vi "AgKs_SpecAn_Capture.vi"(5 "Error In":errorcluster) -> (19 "Error Out":errorcluster)   [LabVIEW 2015]
doc: "AgKs SpecAn Screen Capture is a simple screen capture tool for most Agilent PSA/ESA and Keysight MXA/PXA spectrum analyzers"
uses:
  Controls/FGV Action SpecAn Model.ctl
  Controls/SpecAn Cluster.ctl
panel:
  in  "Noise Source":bool
  in  "Frequency Ref In":i32(ring) items=["Internal", "External"]
  in  "Marker Peak":bool
  in  "Cont Update":bool
  in  "Preamp State":bool
  in  "Avg State":bool
  in  "VBW Auto/Man":bool=TRUE
  in  "RBW Auto/Man":bool=TRUE
  in  "RBW (Hz)":i32=30000000 min=10 step=1 format="%#.6p"
  in  "VBW (Hz)":i32=30000000 min=10 step=1 format="%#.6p"
  in  "Avg Count":u32=10 min=1 max=5000 step=1
  in  "Ref Level (dBm)":dbl=10.0 min=-120.0 max=30.0 step=1.0 format="%#.2f"
  in  "Span (Hz)":dbl=5000000.0 min=10.0 max=30000000000.0 step=1.0 format="%#.6p"
  in  "Center Freq (Hz)":dbl=1000000000.0 min=10.0 max=30000000000.0 step=1.0 format="%#.6p"
  in  "Attenuation (dB)":dbl=20.0 format="%#.2f"
  in  "VISA Handle":refnum<visa-resource-name>="SpecAn"
  in  "Capture":bool
  in  "Auto Align Enable":bool
  in  "Zoom Factor":sgl min=0 max=10 step=0.1
  in  "Secured View":bool
  in  "Full Screen":bool
  out "Pic":picture
  out "PIC_PATH":path
  out "INI PATH":path
  out "State":string="Close GUI"
  out "ZoomFactor_Hi":dbl
  out "ZoomFactor_Lo":dbl
  in  "Save Image?":bool
  # "Note:\n\nPSA screen dim: 640x480\nPSA: Use Zoom Factor = 0\n\nPXA screen dim: 1024x768\nPXA: Use Zoom Factor = 0.7"
  # "Agilent/Keysight PSA/ESA/MXA/PXA Screen Capture Tool"
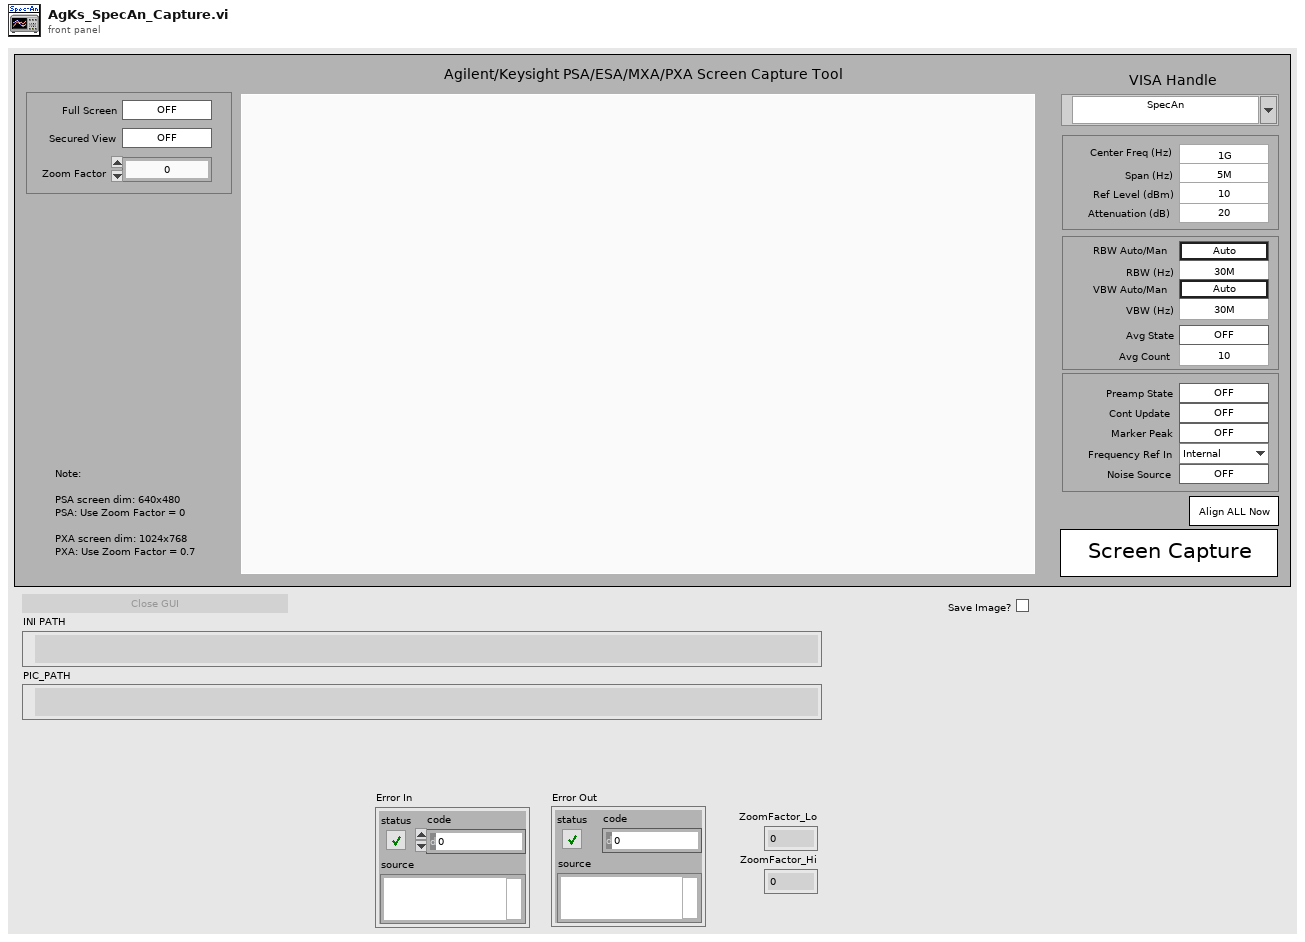
[diagram p1: front panel]
types:
  T1 = cluster{"SA VISA":refnum<visa-resource-name>, "PATH":path, "This VI":refnum<vi>, "VI Name":string}
  T2 = typedef "SpecAn Cluster.ctl" = cluster{"Span (Hz)":dbl, "Center Freq (Hz)":dbl, "Mode":i32, "Frequency Ref In":i32, "Trace Type":i32, "Trace":i32, "Enable Trace Update":bool, "Enable Trace Display":bool, "Manual VBW":i32, "Auto VBW":bool, "Manual RBW":i32, "Auto RBW":bool, "Amplitude Units":i32, "Reference Level":dbl, "Reference Level Offset":dbl, "Averaging On/Off":i32, "Marker Type":i32, "Readout":i32, "Active Marker":i32, "Auto Align Enable":enum16{"Disable", "Enable"}}
  T3 = typedef "FGV Action SpecAn Model.ctl" = enum16{"Get", "Set"}
  T4 = typedef "imagedata.ctl" = cluster{"image type":i32, "image depth":i32, "image":u8[], "mask":u8[], "colors":u32[], "Rectangle":cluster{"left":i16, "top":i16, "right":i16, "bottom":i16}}
  T5 = typedef "SpecAn Model.ctl" = enum16{"E4440", "N9030"}
  T6 = enum32{"Invalid", "Standard", "Closed", "Hidden", "Minimized", "Maximized"}
  T7 = enum32{"invalid app kind", "Development System", "Run Time System", "Student Edition", "Embedded LabVIEW", "Evaluation", "Custom"}
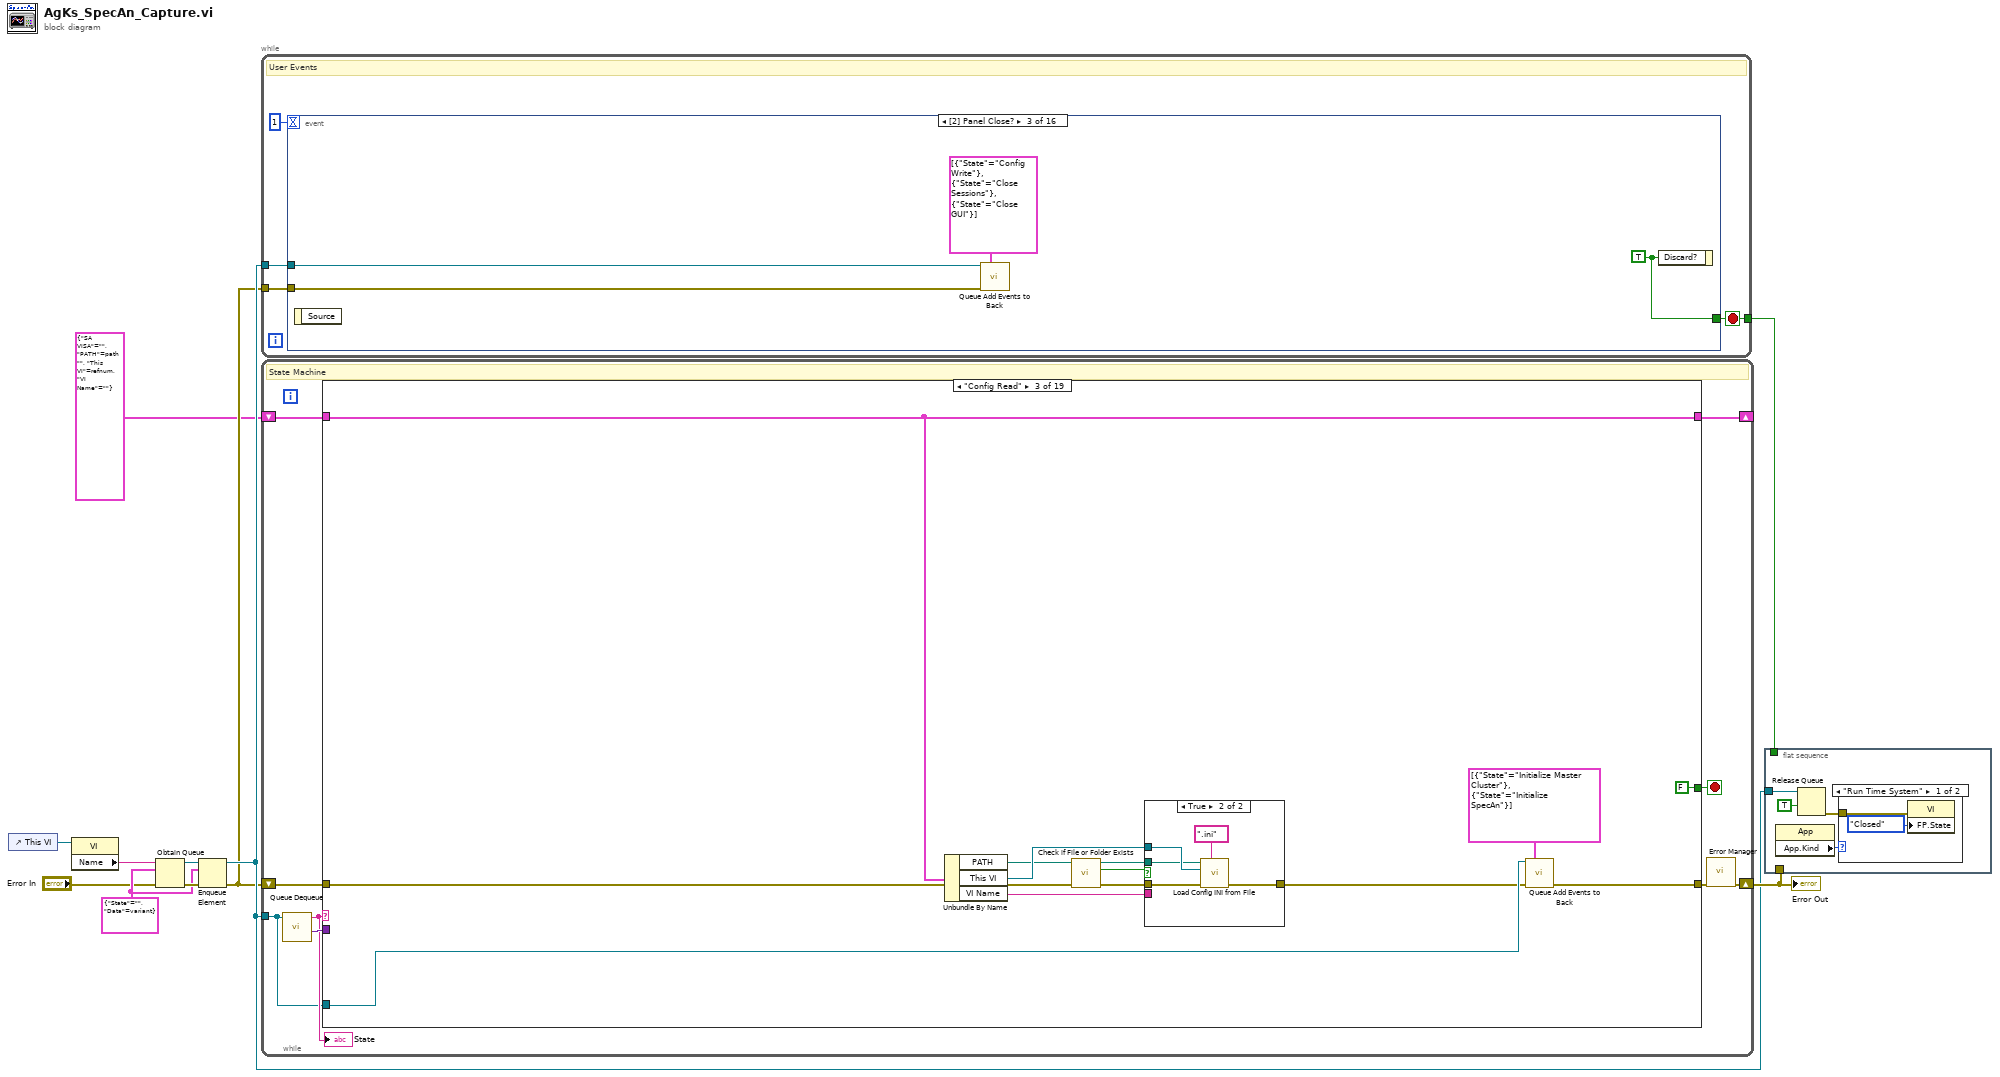
[diagram p0: block diagram]
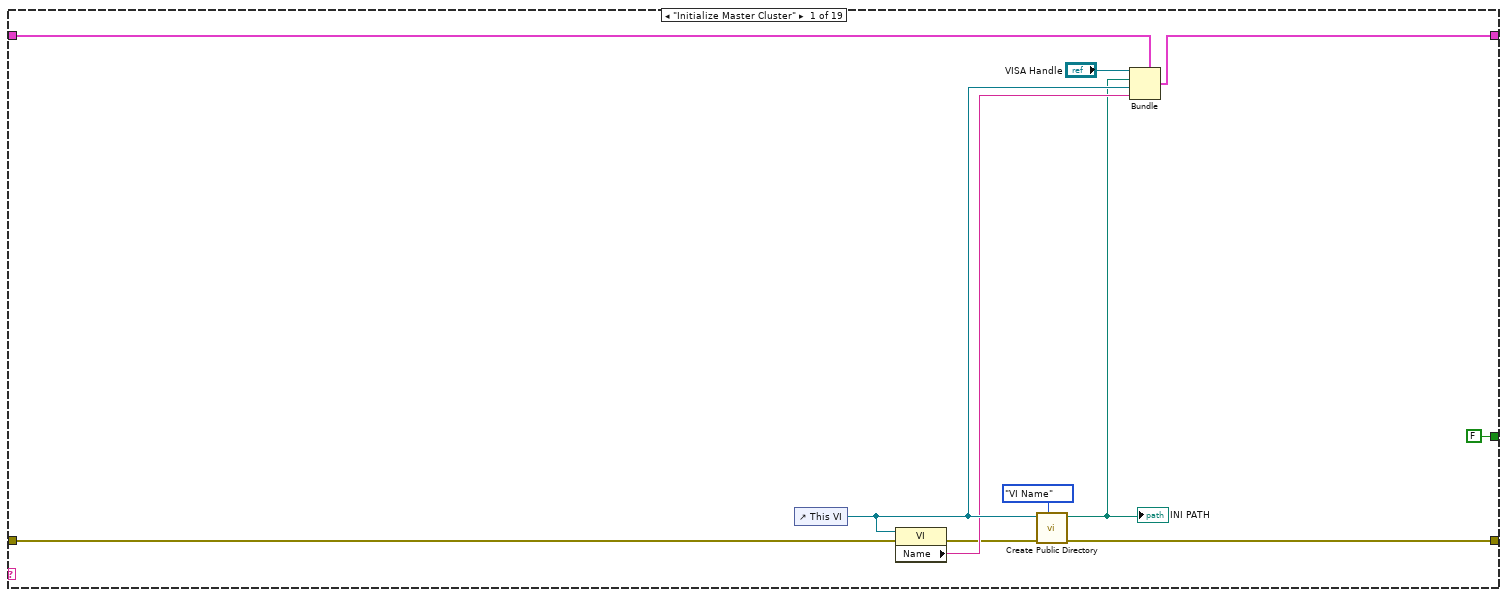
[diagram p3: hidden frame]
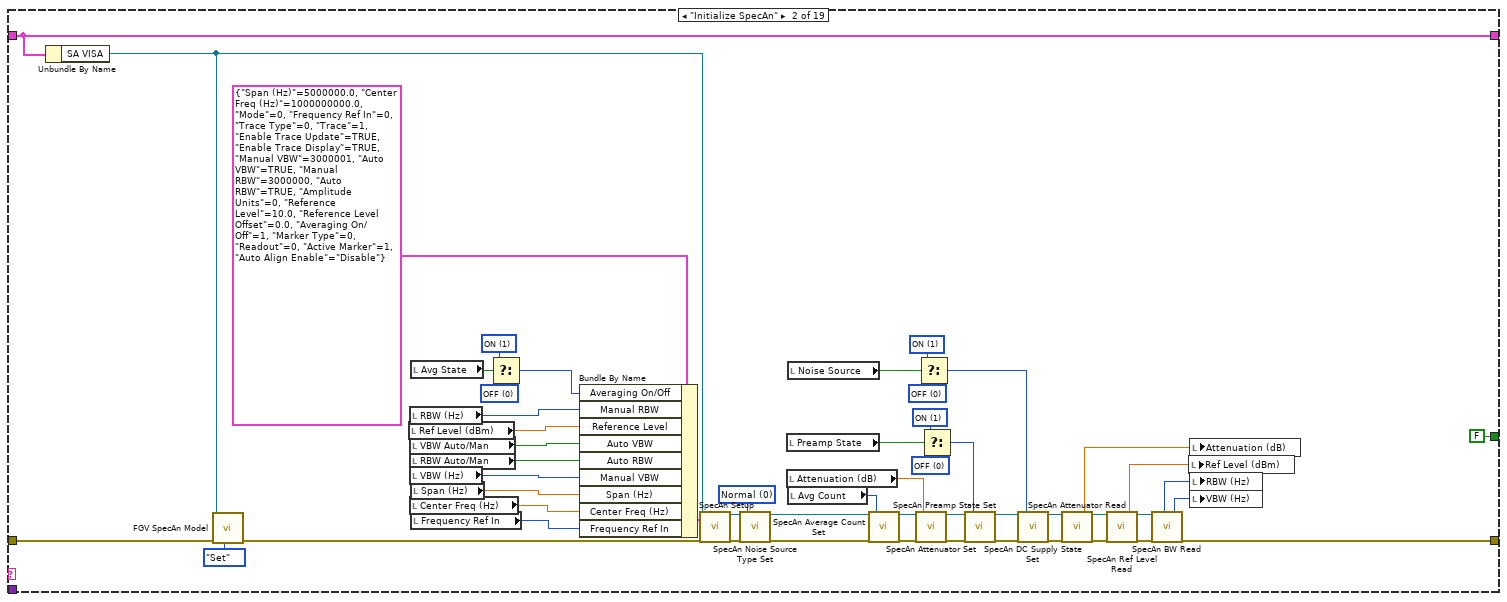
[diagram p4: hidden frame]
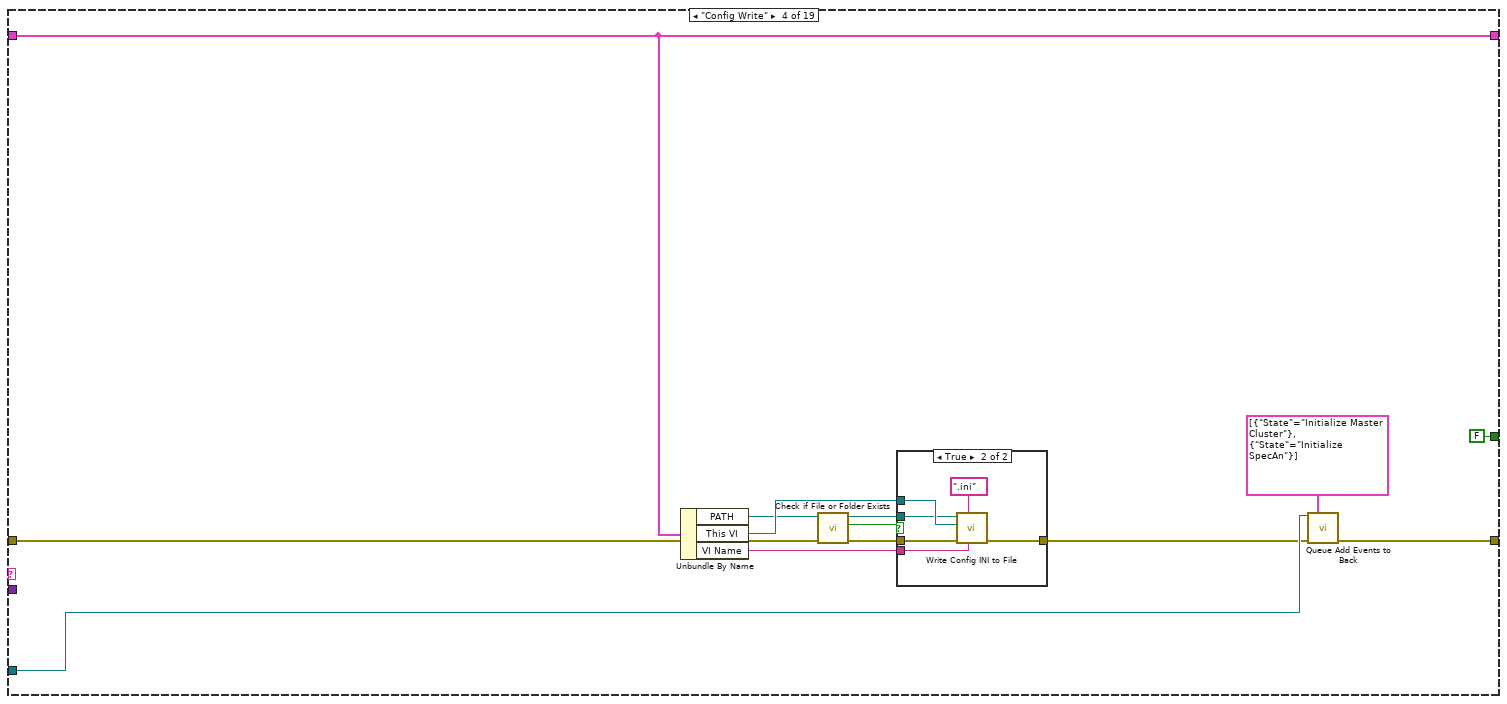
[diagram p6: hidden frame]
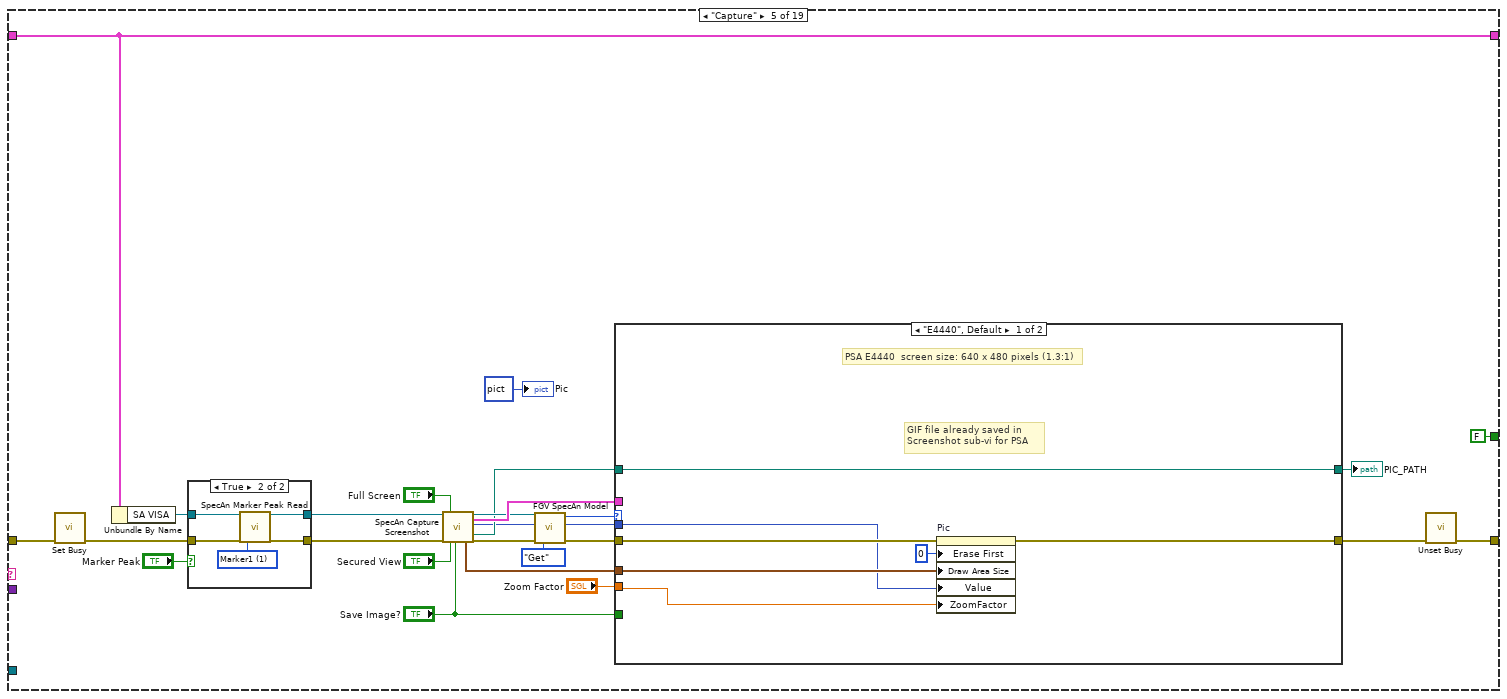
[diagram p8: hidden frame]
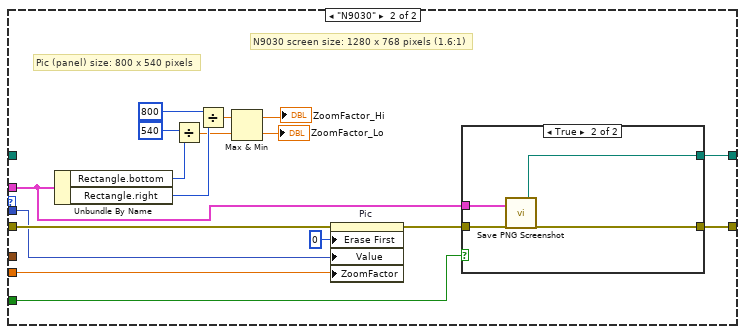
[diagram p9: hidden frame]
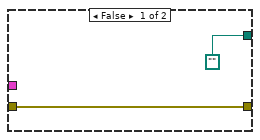
[diagram p10: hidden frame]
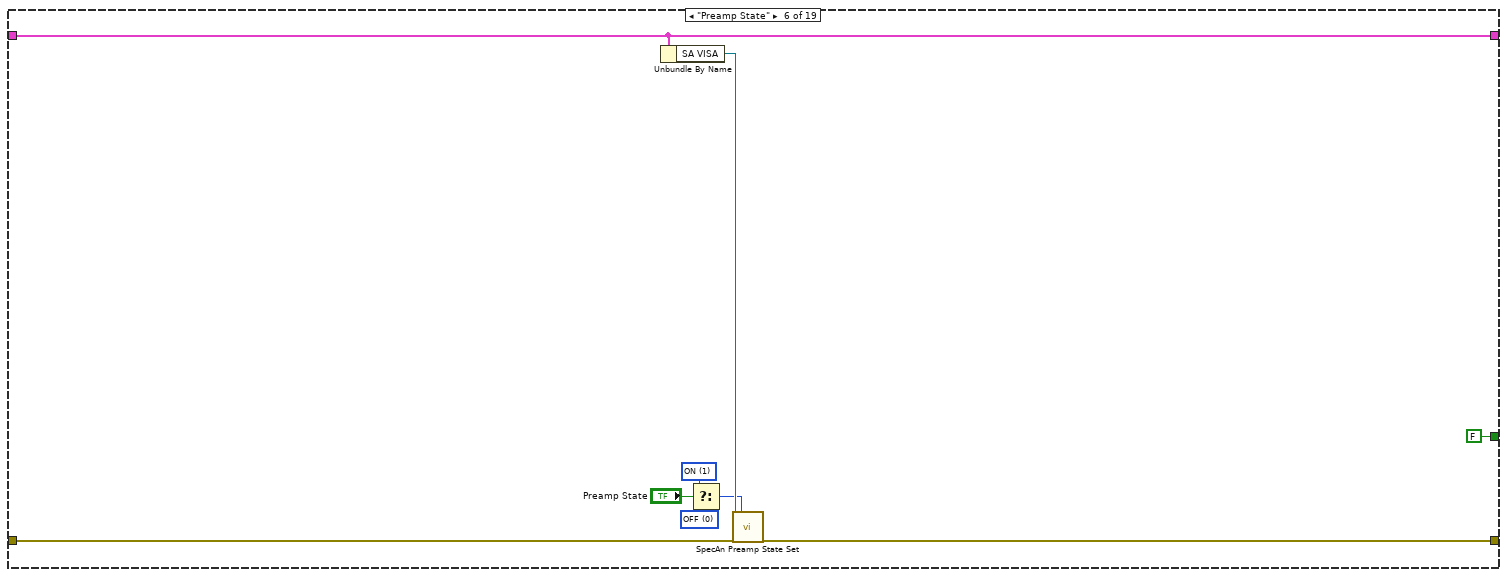
[diagram p12: hidden frame]
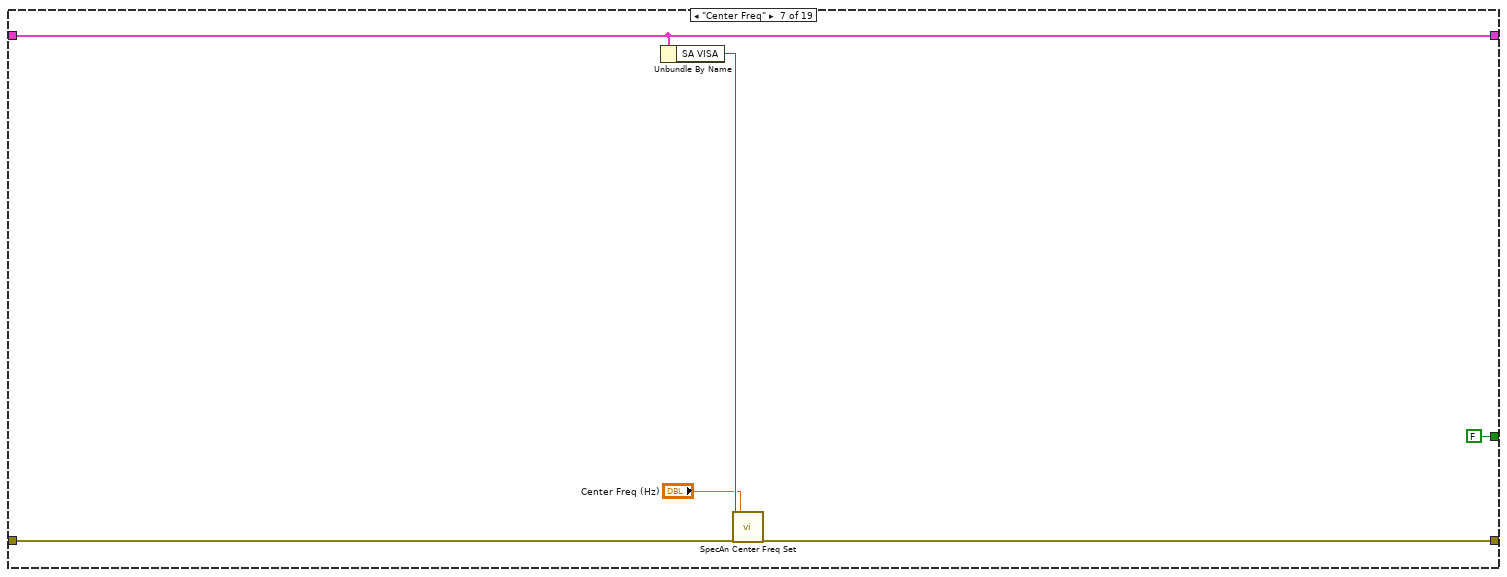
[diagram p13: hidden frame]
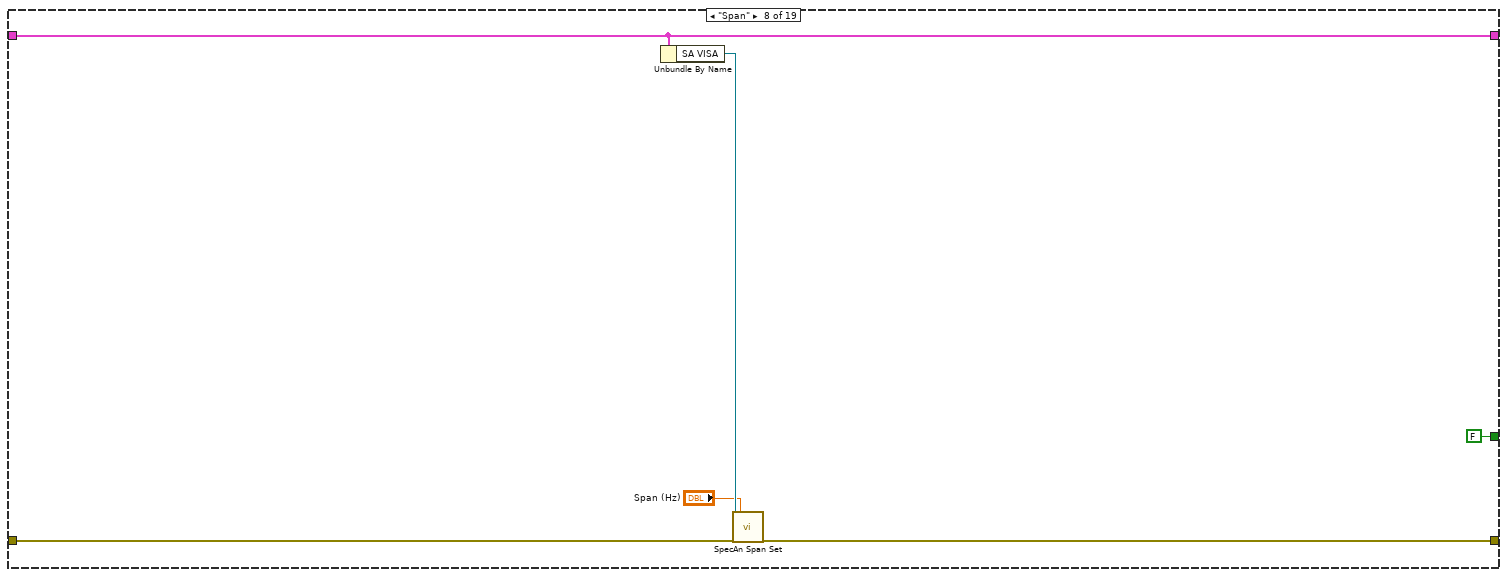
[diagram p14: hidden frame]
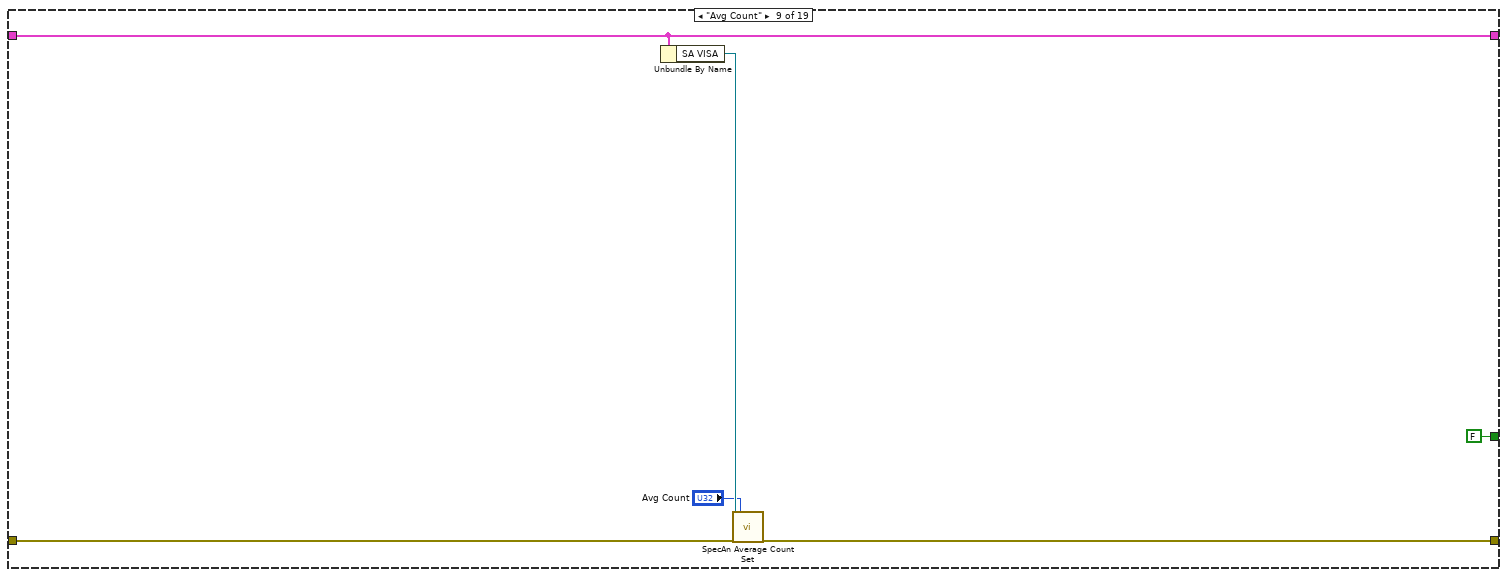
[diagram p15: hidden frame]
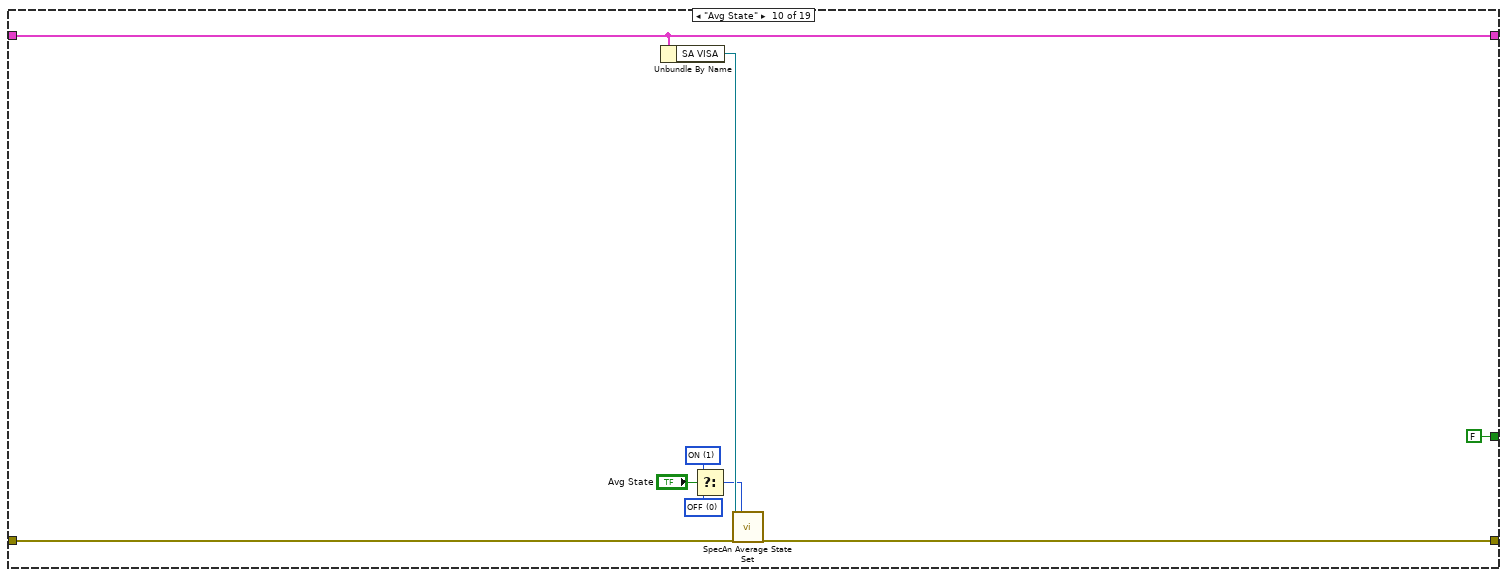
[diagram p16: hidden frame]
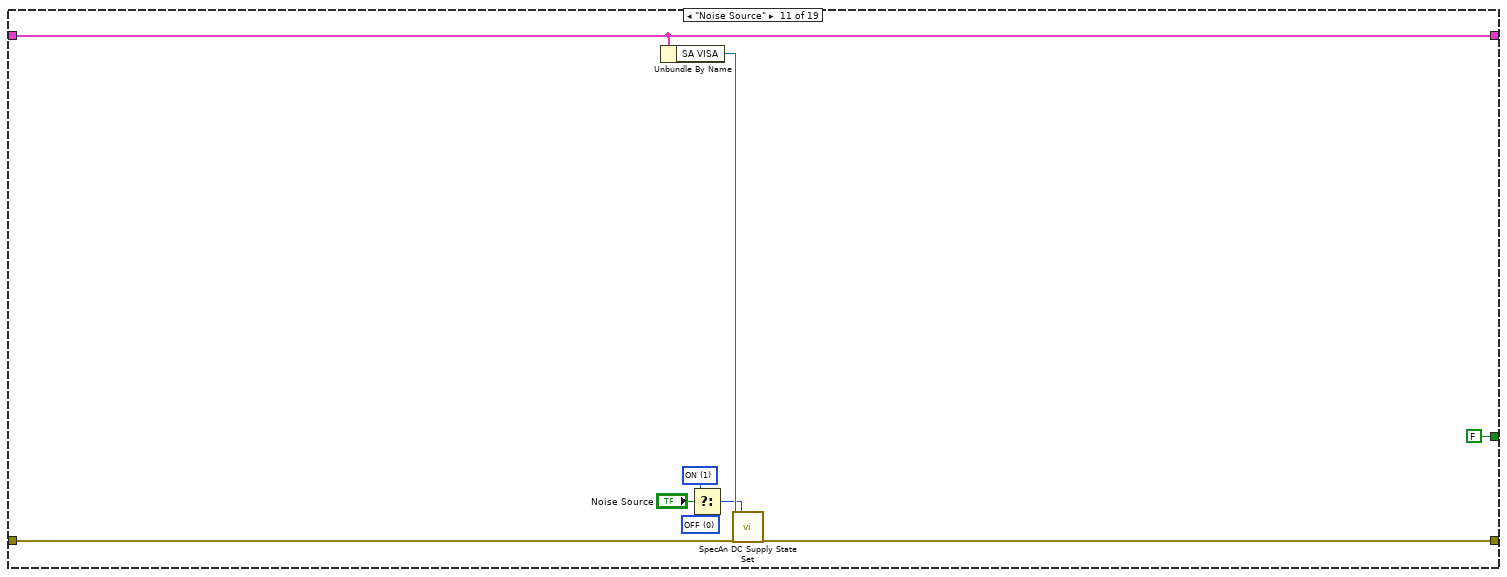
[diagram p17: hidden frame]
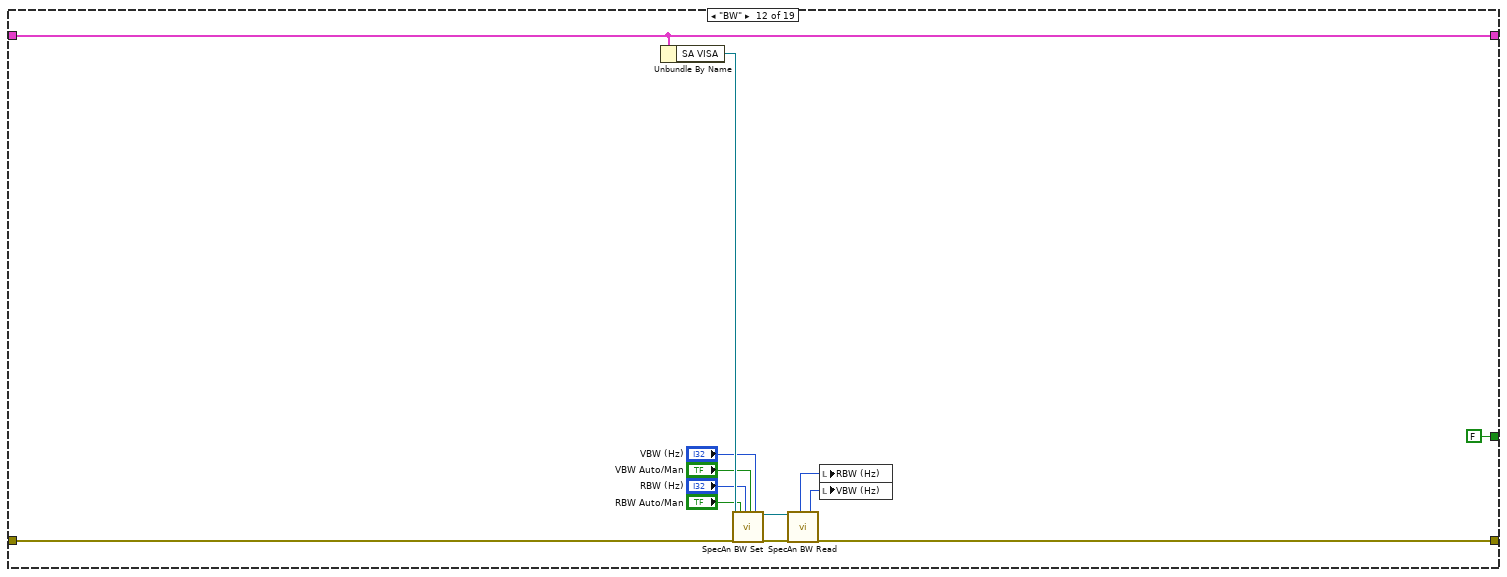
[diagram p18: hidden frame]
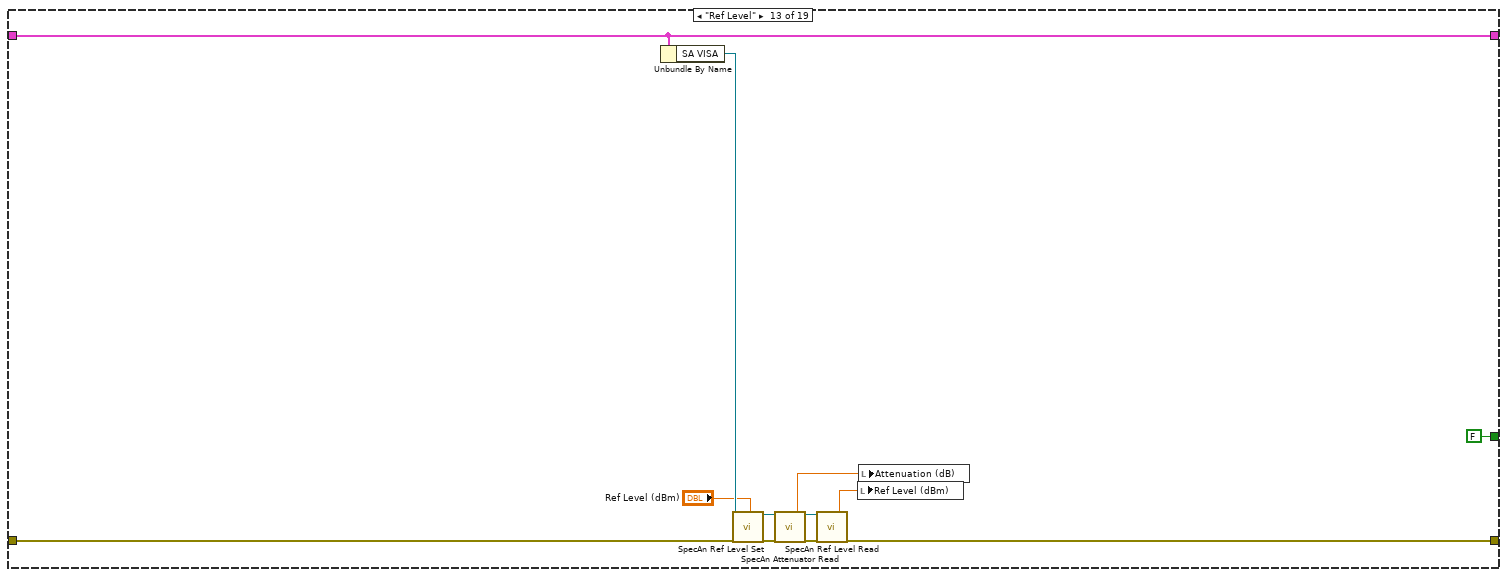
[diagram p19: hidden frame]
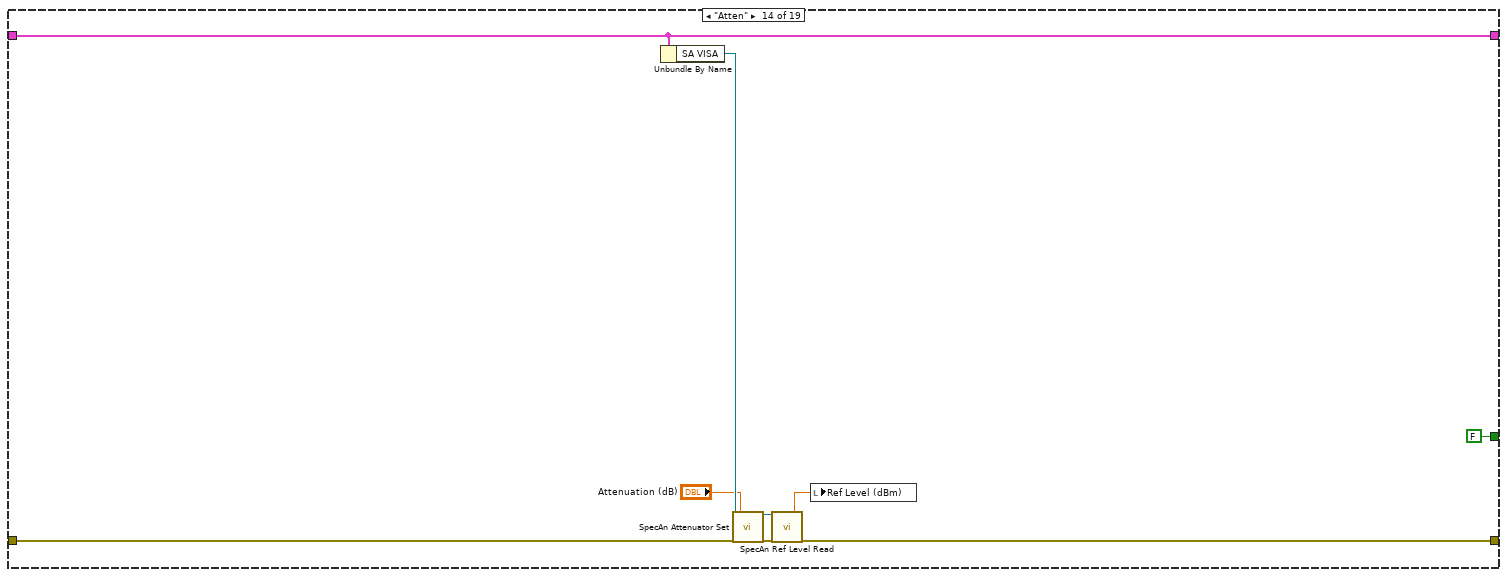
[diagram p20: hidden frame]
diagram:
  w7 = cluster{"State":string, "Data":variant} {"State"="", "Data"=variant} ("Cluster")
  n1 = control-ref of="This VI"() -> (w4:refnum<vi>)
  n2 = property class="VI"(reference=w4) -> ("Name"=w1:string)  [unwired: 1 in, 2 out]
  n3 = Obtain Queue(name (unnamed)=w1, element data type=w7, error in (no error)="Error In") -> (queue out=w10:refnum<queue>, error out=w11:errorcluster)  [unwired: 2 in, 1 out]
  n4 = Enqueue Element(queue=w10, element=w7, error in (no error)=w11) -> (queue out=w6:refnum<queue>, error out=w3:errorcluster)  [unwired: 1 in, 1 out]
  n5 = while {
    tunnel: w6 -> [w15]
    tunnel: [w14] -> w9
    tunnel: w3 -> [w12]
    stop <- w14 stop-if-true
    # "User Events"
    n6 = event shown="[2] Panel Close?" {
      selector: _ -> [_ _ _ _ _ _ _ _ _ _ _ _ _ _ _ _]
      dyn-events: _ -> [_ _ _ _ _ _ _ _ _ _ _ _ _ _ _ _]
      timeout: 1 -> [_ _ _ _ _ _ _ _ _ _ _ _ _ _ _ _]
      tunnel: w15 -> [w18 w25 w33 w36 w39 w42 w45 w48 w51 w54 w57 w60 w63 w66 w69 w72]
      tunnel: [FALSE ("Abort?") FALSE ("Abort?") w32 _ _ _ _ _ _ _ _ _ _ _ _ _] -> w14
      tunnel: w12 -> [w17 w23 w31 w35 w38 w41 w44 w47 w50 w53 w56 w59 w62 w65 w68 _]
      event Timeout {
        n7 = event-data() -> ()  [unwired: 1 in, 1 out]
        n8 = First Call?() -> (First Call?: T/F=w16:bool)
        n9 = case shown="True" w16 {
          tunnel: w18 -> [_ w21]
          tunnel: w17 -> [_ w20]
          frame False {
          }
          frame True {
            n10 = call "Queue Add Events to Back.vi"("Queue In"=w21, "State Array"=cluster{"State":string}[] [{"State"="Config Read"}], "Error In"=w20) -> ()  [unwired: 11 in, 2 out]
          }
        }
      }
      event Menu Selection (User) {
        n11 = event-data() -> ("ItemTag"=w27:string, "ItemPath"=w26:string)  [unwired: 1 in]
        n12 = case shown="Default" w26 {
          tunnel: w25 -> [w30]
          tunnel: w27 -> [w29]
          tunnel: w23 -> [w28]
          frame Default {
            n13 = call "Queue Add Events to Back with Data.vi"("Queue In"=w30, "Error In"=w28, "State"=w29) -> ()  [unwired: 15 in, 2 out]
          }
        }
      }
      event Panel Close? {
        w32 = TRUE ("Discard?")
        n14 = event-data() -> ()  [unwired: 1 in, 1 out]
        n15 = call "Queue Add Events to Back.vi"("Queue In"=w33, "State Array"=cluster{"State":string}[] [{"State"="Config Write"}, {"State"="Close Sessions"}, {"State"="Close GUI"}], "Error In"=w31) -> ()  [unwired: 11 in, 2 out]
        n16 = event-data("Discard?"=w32) -> ()  [unwired: 1 in, 1 out]
      }
      event "VISA Handle": Value Change {
        n17 = event-data() -> ()  [unwired: 1 in, 2 out]
        n18 = call "Queue Add Events to Back.vi"("Queue In"=w36, "State Array"=cluster{"State":string}[] [{"State"="Close Sessions"}, {"State"="Master Cluster"}], "Error In"=w35) -> ()  [unwired: 11 in, 2 out]
      }
      event "Preamp State": Value Change {
        n19 = event-data() -> ()  [unwired: 1 in, 2 out]
        n20 = call "Queue Add Events to Back.vi"("Queue In"=w39, "State Array"=cluster{"State":string}[] [{"State"="Preamp State"}], "Error In"=w38) -> ()  [unwired: 11 in, 2 out]
      }
      event "Center Freq (Hz)": Value Change {
        n21 = event-data() -> ()  [unwired: 1 in, 2 out]
        n22 = call "Queue Add Events to Back.vi"("Queue In"=w42, "State Array"=cluster{"State":string}[] [{"State"="Center Freq"}], "Error In"=w41) -> ()  [unwired: 11 in, 2 out]
      }
      event "Span (Hz)": Value Change {
        n23 = event-data() -> ()  [unwired: 1 in, 2 out]
        n24 = call "Queue Add Events to Back.vi"("Queue In"=w45, "State Array"=cluster{"State":string}[] [{"State"="Span"}], "Error In"=w44) -> ()  [unwired: 11 in, 2 out]
      }
      event "Avg Count": Value Change {
        n25 = event-data() -> ()  [unwired: 1 in, 2 out]
        n26 = call "Queue Add Events to Back.vi"("Queue In"=w48, "State Array"=cluster{"State":string}[] [{"State"="Avg Count"}], "Error In"=w47) -> ()  [unwired: 11 in, 2 out]
      }
      event "Avg State": Value Change {
        n27 = event-data() -> ()  [unwired: 1 in, 2 out]
        n28 = call "Queue Add Events to Back.vi"("Queue In"=w51, "State Array"=cluster{"State":string}[] [{"State"="Avg State"}], "Error In"=w50) -> ()  [unwired: 11 in, 2 out]
      }
      event "VBW (Hz)", "VBW Auto/Man", "RBW (Hz)", "RBW Auto/Man": Value Change {
        n29 = event-data() -> ()  [unwired: 1 in, 2 out]
        n30 = call "Queue Add Events to Back.vi"("Queue In"=w54, "State Array"=cluster{"State":string}[] [{"State"="BW"}], "Error In"=w53) -> ()  [unwired: 11 in, 2 out]
      }
      event "Ref Level (dBm)": Value Change {
        n31 = event-data() -> ()  [unwired: 1 in, 2 out]
        n32 = call "Queue Add Events to Back.vi"("Queue In"=w57, "State Array"=cluster{"State":string}[] [{"State"="Ref Level"}], "Error In"=w56) -> ()  [unwired: 11 in, 2 out]
      }
      event "Attenuation (dB)": Value Change {
        n33 = event-data() -> ()  [unwired: 1 in, 2 out]
        n34 = call "Queue Add Events to Back.vi"("Queue In"=w60, "State Array"=cluster{"State":string}[] [{"State"="Atten"}], "Error In"=w59) -> ()  [unwired: 11 in, 2 out]
      }
      event "Frequency Ref In": Value Change {
        n35 = event-data() -> ()  [unwired: 1 in, 2 out]
        n36 = call "Queue Add Events to Back.vi"("Queue In"=w63, "State Array"=cluster{"State":string}[] [{"State"="Freq Ref"}], "Error In"=w62) -> ()  [unwired: 11 in, 2 out]
      }
      event "Auto Align Enable": Value Change {
        n37 = event-data() -> ()  [unwired: 1 in, 2 out]
        n38 = call "Queue Add Events to Back.vi"("Queue In"=w66, "State Array"=cluster{"State":string}[] [{"State"="Auto Align"}], "Error In"=w65) -> ()  [unwired: 11 in, 2 out]
      }
      event "Noise Source": Value Change {
        n39 = event-data() -> ()  [unwired: 1 in, 2 out]
        n40 = call "Queue Add Events to Back.vi"("Queue In"=w69, "State Array"=cluster{"State":string}[] [{"State"="Noise Source"}], "Error In"=w68) -> ()  [unwired: 11 in, 2 out]
      }
      event "Capture": Value Change {
        n41 = event-data() -> ("NewVal"=w71:bool)  [unwired: 1 in]
        n42 = case shown="True" w71 {
          tunnel: w72 -> [_ w73]
          frame False {
          }
          frame True {
            n43 = call "Queue Add Events to Back.vi"("Queue In"=w73, "State Array"=cluster{"State":string}[] [{"State"="Capture"}]) -> ()  [unwired: 12 in, 2 out]
          }
        }
      }
    }
  }
  n44 = while {
    shift-right: [w83] -> w8
    shift-left: w3 -> [w75]
    shift-right: [w79] -> _
    shift-left: T1 {"SA VISA"="", "PATH"=path "", "This VI"=refnum, "VI Name"=""} -> [w80]
    tunnel: w6 -> [w76]
    stop <- w81 stop-if-true
    # "State Machine"
    n45 = call "Queue Dequeue.vi"("Queue In"=w76) -> ("Data"=w78:variant, "State"=w77:string)  [unwired: 8 in, 1 out]
    "State" <- w77
    n46 = case shown="\"Config Read\"" w77 {
      tunnel: [w91 w144 w158 w177 w187 w248 w259 w265 w271 w280 w289 w296 w307 w319 w329 w334 w348 w358 w364] -> w82
      tunnel: w76 -> [_ _ w159 w178 _ _ _ _ _ _ _ _ _ _ _ _ w347 _ _]
      tunnel: [FALSE FALSE FALSE FALSE FALSE FALSE FALSE FALSE FALSE FALSE FALSE FALSE FALSE FALSE FALSE FALSE FALSE FALSE TRUE] -> w81
      tunnel: w80 -> [w92 w96 w154 w173 w209 w254 w261 w267 w273 w282 w291 w304 w316 w325 w332 w338 w350 w361 w362]
      tunnel: [w94 w96 w154 w173 w209 w254 w261 w267 w273 w282 w291 w304 w316 w325 w332 w338 w350 w361 w362] -> w79
      tunnel: w78 -> [_ _ _ _ _ _ _ _ _ _ _ _ _ _ _ _ _ _ _]
      tunnel: w75 -> [w85 w145 w151 w170 w203 w255 w260 w266 w272 w281 w290 w303 w315 w323 w330 w337 w349 w360 w364]
      frame "Initialize Master Cluster" {
        n47 = control-ref of="This VI"() -> (w90:refnum<vi>)
        n48 = property class="VI"(reference=w90, error in=w85) -> (error out=w84:errorcluster, "Name"=w89:string)  [unwired: 1 out]
        n49 = call "Create Public Directory.vi"("Name Type"=enum16{"VI Name", "Custom Name"}."VI Name", "error in (no error)"=w84, "Caller_VI"=w90) -> ("error out"=w91:errorcluster, "PATH"=w87:path)  [unwired: 7 in]
        "INI PATH" <- w87
        n50 = Bundle(cluster=w92, "SA VISA"="VISA Handle", "PATH"=w87, "This VI"=w90, "VI Name"=w89) -> (w94:T1)
      }
      frame "Initialize SpecAn" {
        w104 = 0 items=["OFF", "ON"] ("State")
        w103 = 1 items=["OFF", "ON"] ("State")
        w109 = 0 items=["Normal", "SNS"] ("Type")
        w128 = 0 items=["OFF", "ON"] ("Averaging On/Off")
        w127 = 1 items=["OFF", "ON"] ("Averaging On/Off")
        w131 = 1 items=["OFF", "ON"] ("State")
        w132 = 0 items=["OFF", "ON"] ("State")
        n51 = Unbundle By Name(w96) -> ("SA VISA"=w95:refnum<visa-resource-name>)
        n52 = call "FGV SpecAn Model.vi"("Action"=FGV_Action_SpecAn_Model."Set", "Error In"=w145, "VISA In"=w95) -> ("Error Out"=w138:errorcluster)  [unwired: 4 in, 1 out]
        n53 = local read "Ref Level (dBm)"() -> (w125:dbl)
        n54 = local read "RBW (Hz)"() -> (w119:i32)
        n55 = local read "VBW Auto/Man"() -> (w124:bool)
        n56 = local read "RBW Auto/Man"() -> (w123:bool)
        n57 = local read "VBW (Hz)"() -> (w120:i32)
        n58 = local read "Center Freq (Hz)"() -> (w121:dbl)
        n59 = local read "Avg State"() -> (w129:bool)
        n60 = local read "Span (Hz)"() -> (w122:dbl)
        n61 = local read "Frequency Ref In"() -> (w110:i32)
        n62 = Select(t=w127, s=w129, f=w128) -> (s? t:f=w126:i32)
        n63 = Bundle By Name(cluster=T2 {"Span (Hz)"=5000000.0, "Center Freq (Hz)"=1000000000.0, "Mode"=0, "Frequency Ref In"=0, "Trace Type"=0, "Trace"=1, "Enable Trace Update"=TRUE, "Enable Trace Display"=TRUE, "Manual VBW"=3000001, "Auto VBW"=TRUE, "Manual RBW"=3000000, "Auto RBW"=TRUE, "Amplitude Units"=0, "Reference Level"=10.0, "Reference Level Offset"=0.0, "Averaging On/Off"=1, "Marker Type"=0, "Readout"=0, "Active Marker"=1, "Auto Align Enable"=enum."Disable"} ("SpecAn Cluster"), "Averaging On/Off"=w126, "Manual RBW"=w119, "Reference Level"=w125, "Auto VBW"=w124, "Auto RBW"=w123, "Manual VBW"=w120, "Span (Hz)"=w122, "Center Freq (Hz)"=w121, "Frequency Ref In"=w110) -> (w141:T2)
        n64 = call "SpecAn Setup.vi"("VISA In"=w95, "SpecAn Cluster"=w141, "Error In"=w138) -> ("VISA Out"=w106:refnum<visa-resource-name>, "Error Out"=w108:errorcluster)  [unwired: 15 in]
        n65 = call "SpecAn Noise Source Type Set.vi"("VISA In"=w106, "Error In"=w108, "Type"=w109) -> ("VISA Out"=w105:refnum<visa-resource-name>, "Error Out"=w107:errorcluster)  [unwired: 15 in]
        n66 = local read "Preamp State"() -> (w133:bool)
        n67 = local read "Attenuation (dB)"() -> (w134:dbl)
        n68 = local read "Noise Source"() -> (w102:bool)
        n69 = local read "Avg Count"() -> (w135:u32)
        n70 = call "SpecAn Average Count Set.vi"("VISA In"=w105, "Error In"=w107, "Avg Count"=w135) -> ("VISA Out"=w139:refnum<visa-resource-name>, "Error Out"=w140:errorcluster)  [unwired: 15 in]
        n71 = call "SpecAn Attenuator Set.vi"("VISA In"=w139, "Error In"=w140, "Attenuation (dB)"=w134) -> ("VISA Out"=w136:refnum<visa-resource-name>, "Error Out"=w137:errorcluster)  [unwired: 15 in]
        n72 = Select(t=w103, s=w102, f=w104) -> (s? t:f=w101:i32)
        n73 = Select(t=w131, s=w133, f=w132) -> (s? t:f=w130:i32)
        n74 = call "SpecAn Preamp State Set.vi"("VISA In"=w136, "Error In"=w137, "State"=w130) -> ("VISA Out"=w100:refnum<visa-resource-name>, "Error Out"=w97:errorcluster)  [unwired: 15 in]
        n75 = call "SpecAn DC Supply State Set.vi"("VISA In"=w100, "Error In"=w97, "State"=w101) -> ("VISA Out"=w99:refnum<visa-resource-name>, "Error Out"=w98:errorcluster)  [unwired: 15 in]
        n76 = call "SpecAn Attenuator Read.vi"("VISA In"=w99, "Error In"=w98) -> ("Attenuation (dB)"=w112:dbl, "VISA Out"=w113:refnum<visa-resource-name>, "Error Out"=w116:errorcluster)  [unwired: 15 in]
        n77 = call "SpecAn Ref Level Read.vi"("VISA In"=w113, "Error In"=w116) -> ("Ref Level (dBm)"=w111:dbl, "VISA Out"=w114:refnum<visa-resource-name>, "Error Out"=w115:errorcluster)  [unwired: 15 in]
        n78 = call "SpecAn BW Read.vi"("VISA In"=w114, "Error In"=w115) -> ("Manual RBW"=w118:i32, "Manual VBW"=w117:i32, "Error Out"=w144:errorcluster)  [unwired: 12 in, 3 out]
        n79 = local write "Ref Level (dBm)"(w111) -> ()
        n80 = local write "Attenuation (dB)"(w112) -> ()
        n81 = local write "RBW (Hz)"(w118) -> ()
        n82 = local write "VBW (Hz)"(w117) -> ()
      }
      frame "Config Read" {
        n83 = Unbundle By Name(w154) -> ("PATH"=w149:path, "This VI"=w153:refnum<vi>, "VI Name"=w152:string)
        n84 = call <vilib>:"Check if File or Folder Exists.vi"("error in (no error)"=w151, "path"=w149) -> ("error out"=w150:errorcluster, "file or folder exists?"=w147:bool, "dup path"=w148:path)  [unwired: 7 in]
        n85 = case shown="True" w147 {
          tunnel: w150 -> [w160 w165]
          tunnel: [w160 w164] -> w155
          tunnel: w153 -> [_ w162]
          tunnel: w152 -> [_ _]
          tunnel: w148 -> [_ w161]
          frame False {
          }
          frame True {
            n86 = call "Load Config INI from File.vi"("File Type"=".ini", "Error In"=w165, "reference"=w162, "Path In"=w161) -> ("Error Out"=w164:errorcluster)  [unwired: 6 in, 1 out]
          }
        }
        n87 = call "Queue Add Events to Back.vi"("Queue In"=w159, "State Array"=cluster{"State":string}[] [{"State"="Initialize Master Cluster"}, {"State"="Initialize SpecAn"}], "Error In"=w155) -> ("Error Out"=w158:errorcluster)  [unwired: 11 in, 1 out]
      }
      frame "Config Write" {
        n88 = Unbundle By Name(w173) -> ("PATH"=w168:path, "This VI"=w172:refnum<vi>, "VI Name"=w171:string)
        n89 = call <vilib>:"Check if File or Folder Exists.vi"("error in (no error)"=w170, "path"=w168) -> ("error out"=w169:errorcluster, "file or folder exists?"=w166:bool, "dup path"=w167:path)  [unwired: 7 in]
        n90 = case shown="True" w166 {
          tunnel: w169 -> [w179 w185]
          tunnel: [w179 w184] -> w174
          tunnel: w172 -> [_ w182]
          tunnel: w171 -> [_ w181]
          tunnel: w167 -> [_ w180]
          frame False {
          }
          frame True {
            n91 = call "Write Config INI to File.vi"("File Name"=w181, "File Type"=".ini", "Error In"=w185, "reference"=w182, "Path In"=w180) -> ("Error Out"=w184:errorcluster)  [unwired: 5 in, 1 out]
          }
        }
        n92 = call "Queue Add Events to Back.vi"("Queue In"=w178, "State Array"=cluster{"State":string}[] [{"State"="Initialize Master Cluster"}, {"State"="Initialize SpecAn"}], "Error In"=w174) -> ("Error Out"=w177:errorcluster)  [unwired: 11 in, 1 out]
      }
      frame "Capture" {
        n93 = call <vilib>:"Set Busy.vi"("error in (no error)"=w203) -> ("error out"=w188:errorcluster)  [unwired: 9 in, 1 out]
        n94 = Unbundle By Name(w209) -> ("SA VISA"=w206:refnum<visa-resource-name>)
        n95 = case shown="True" "Marker Peak" {
          tunnel: w206 -> [w241 w247]
          tunnel: [w241 w246] -> w205
          tunnel: [w242 w245] -> w204
          tunnel: w188 -> [w242 w244]
          frame False {
          }
          frame True {
            w243 = 1 items=["Marker1"=1, "Marker2"=2, "Marker3"=3, "Marker4"=4, "Marker5"=5, "Marker6"=6, "Marker7"=7, "Marker8"=8, "Marker9"=9, "Marker10"=10, "Marker11"=11, "Marker12"=12] ("Active Marker")
            n96 = call "SpecAn Marker Peak Read.vi"("VISA In"=w247, "Error In"=w244, "Active Marker"=w243) -> ("VISA Out"=w246:refnum<visa-resource-name>, "Error Out"=w245:errorcluster)  [unwired: 13 in, 2 out]
          }
        }
        n97 = call "SpecAn Capture Screenshot.vi"("VISA In"=w205, "Error In"=w204, "Full Screen"="Full Screen", "Secured View"="Secured View", "Save Image?"="Save Image?") -> ("image size"=w193:cluster{"Width":u32, "Height":u32}, "VISA Out"=w195:refnum<visa-resource-name>, "image data"=w208:T4, "Pic"=w191:picture, "GIF_PATH"=w194:path, "Error Out"=w197:errorcluster)  [unwired: 9 in]
        n98 = call "FGV SpecAn Model.vi"("Action"=FGV_Action_SpecAn_Model."Get", "Error In"=w197, "VISA In"=w195) -> ("Error Out"=w196:errorcluster, "SA Model"=w198:T5)  [unwired: 4 in]
        n99 = case shown="\"E4440\", Default" w198 {
          tunnel: w196 -> [w216 w231]
          tunnel: w208 -> [_ w233]
          tunnel: [w215 w234] -> w207
          tunnel: [w217 w232] -> w186
          tunnel: w194 -> [w217 _]
          tunnel: w193 -> [w214 _]
          tunnel: "Zoom Factor" -> [w212 w227]
          tunnel: w191 -> [w211 w229]
          tunnel: "Save Image?" -> [_ w220]
          frame "E4440", Default {
            # "PSA E4440  screen size: 640 x 480 pixels (1.3:1)"
            # "GIF file already saved in\nScreenshot sub-vi for PSA"
            n100 = property on="Pic" class="Pict"(error in=w216, "Erase First"=u8 0, "Draw Area Size"=w214, "Value"=w211, "ZoomFactor"=w212) -> (error out=w215:errorcluster)  [unwired: 1 in, 1 out]
          }
          frame "N9030" {
            # "Pic (panel) size: 800 x 540 pixels"
            # "N9030 screen size: 1280 x 768 pixels (1.6:1)"
            n101 = Unbundle By Name(w233) -> ("Rectangle.bottom"=w225:i16, "Rectangle.right"=w226:i16)
            n102 = Divide(x=i16 540, y=w225) -> (x/y=w224:dbl)
            n103 = Divide(x=i16 800, y=w226) -> (x/y=w223:dbl)
            n104 = Max & Min(x=w223, y=w224) -> (max(x,y)=→"ZoomFactor_Hi":dbl, min(x,y)=→"ZoomFactor_Lo":dbl)
            n105 = property on="Pic" class="Pict"(error in=w231, "Erase First"=u8 0, "Value"=w229, "ZoomFactor"=w227) -> (error out=w230:errorcluster)  [unwired: 1 in, 1 out]
            n106 = case shown="True" w220 {
              tunnel: w230 -> [w236 w240]
              tunnel: w233 -> [_ w239]
              tunnel: [w236 w238] -> w234
              tunnel: [path "" w237] -> w232
              frame False {
              }
              frame True {
                n107 = call "Save PNG Screenshot.vi"("image data"=w239, "Error In"=w240) -> ("Path"=w237:path, "Error Out"=w238:errorcluster)  [unwired: 16 in]
              }
            }
          }
        }
        "PIC_PATH" <- w186
        n108 = call <vilib>:"Unset Busy.vi"("error in (no error)"=w207) -> ("error out"=w187:errorcluster)  [unwired: 10 in]
        "Pic" <- picture data[5B] ("Pic")
      }
      frame "Preamp State" {
        w251 = 1 items=["OFF", "ON"] ("State")
        w252 = 0 items=["OFF", "ON"] ("State")
        n109 = Unbundle By Name(w254) -> ("SA VISA"=w253:refnum<visa-resource-name>)
        n110 = Select(t=w251, s="Preamp State", f=w252) -> (s? t:f=w249:i32)
        n111 = call "SpecAn Preamp State Set.vi"("VISA In"=w253, "Error In"=w255, "State"=w249) -> ("Error Out"=w248:errorcluster)  [unwired: 15 in, 1 out]
      }
      frame "Center Freq" {
        n112 = Unbundle By Name(w261) -> ("SA VISA"=w258:refnum<visa-resource-name>)
        n113 = call "SpecAn Center Freq Set.vi"("VISA In"=w258, "Error In"=w260, "Center Freq (Hz)"="Center Freq (Hz)") -> ("Error Out"=w259:errorcluster)  [unwired: 15 in, 1 out]
      }
      frame "Span" {
        n114 = Unbundle By Name(w267) -> ("SA VISA"=w264:refnum<visa-resource-name>)
        n115 = call "SpecAn Span Set.vi"("VISA In"=w264, "Error In"=w266, "Span (Hz)"="Span (Hz)") -> ("Error Out"=w265:errorcluster)  [unwired: 15 in, 1 out]
      }
      frame "Avg Count" {
        n116 = Unbundle By Name(w273) -> ("SA VISA"=w270:refnum<visa-resource-name>)
        n117 = call "SpecAn Average Count Set.vi"("VISA In"=w270, "Error In"=w272, "Avg Count"="Avg Count") -> ("Error Out"=w271:errorcluster)  [unwired: 15 in, 1 out]
      }
      frame "Avg State" {
        w276 = 1 items=["OFF", "ON"] ("Averaging On/Off")
        w277 = 0 items=["OFF", "ON"] ("Averaging On/Off")
        n118 = Unbundle By Name(w282) -> ("SA VISA"=w279:refnum<visa-resource-name>)
        n119 = Select(t=w276, s="Avg State", f=w277) -> (s? t:f=w275:i32)
        n120 = call "SpecAn Average State Set.vi"("VISA In"=w279, "Error In"=w281, "Averaging On/Off"=w275) -> ("Error Out"=w280:errorcluster)  [unwired: 15 in, 1 out]
      }
      frame "Noise Source" {
        w286 = 0 items=["OFF", "ON"] ("State")
        w285 = 1 items=["OFF", "ON"] ("State")
        n121 = Unbundle By Name(w291) -> ("SA VISA"=w288:refnum<visa-resource-name>)
        n122 = Select(t=w285, s="Noise Source", f=w286) -> (s? t:f=w284:i32)
        n123 = call "SpecAn DC Supply State Set.vi"("VISA In"=w288, "Error In"=w290, "State"=w284) -> ("Error Out"=w289:errorcluster)  [unwired: 15 in, 1 out]
      }
      frame "BW" {
        n124 = Unbundle By Name(w304) -> ("SA VISA"=w302:refnum<visa-resource-name>)
        n125 = call "SpecAn BW Set.vi"("VISA In"=w302, "Error In"=w303, "Auto RBW (T: Enable)"="RBW Auto/Man", "Manual RBW"="RBW (Hz)", "Auto VBW (T: Enable)"="VBW Auto/Man", "Manual VBW"="VBW (Hz)") -> ("VISA Out"=w295:refnum<visa-resource-name>, "Error Out"=w297:errorcluster)  [unwired: 12 in]
        n126 = call "SpecAn BW Read.vi"("VISA In"=w295, "Error In"=w297) -> ("Manual RBW"=w294:i32, "Manual VBW"=w293:i32, "Error Out"=w296:errorcluster)  [unwired: 12 in, 3 out]
        n127 = local write "RBW (Hz)"(w294) -> ()
        n128 = local write "VBW (Hz)"(w293) -> ()
      }
      frame "Ref Level" {
        n129 = Unbundle By Name(w316) -> ("SA VISA"=w314:refnum<visa-resource-name>)
        n130 = call "SpecAn Ref Level Set.vi"("VISA In"=w314, "Error In"=w315, "Reference Level (0 dBm)"="Ref Level (dBm)") -> ("VISA Out"=w311:refnum<visa-resource-name>, "Error Out"=w312:errorcluster)  [unwired: 15 in]
        n131 = call "SpecAn Attenuator Read.vi"("VISA In"=w311, "Error In"=w312) -> ("Attenuation (dB)"=w310:dbl, "VISA Out"=w309:refnum<visa-resource-name>, "Error Out"=w308:errorcluster)  [unwired: 15 in]
        n132 = call "SpecAn Ref Level Read.vi"("VISA In"=w309, "Error In"=w308) -> ("Ref Level (dBm)"=w306:dbl, "Error Out"=w307:errorcluster)  [unwired: 15 in, 1 out]
        n133 = local write "Ref Level (dBm)"(w306) -> ()
        n134 = local write "Attenuation (dB)"(w310) -> ()
      }
      frame "Atten" {
        n135 = Unbundle By Name(w325) -> ("SA VISA"=w324:refnum<visa-resource-name>)
        n136 = call "SpecAn Attenuator Set.vi"("VISA In"=w324, "Error In"=w323, "Attenuation (dB)"="Attenuation (dB)") -> ("VISA Out"=w321:refnum<visa-resource-name>, "Error Out"=w320:errorcluster)  [unwired: 15 in]
        n137 = call "SpecAn Ref Level Read.vi"("VISA In"=w321, "Error In"=w320) -> ("Ref Level (dBm)"=w318:dbl, "Error Out"=w319:errorcluster)  [unwired: 15 in, 1 out]
        n138 = local write "Ref Level (dBm)"(w318) -> ()
      }
      frame "Freq Ref" {
        n139 = Unbundle By Name(w332) -> ("SA VISA"=w331:refnum<visa-resource-name>)
        n140 = call "SpecAn Freq Ref Set.vi"("VISA In"=w331, "Error In"=w330, "Freq Ref"="Frequency Ref In") -> ("Error Out"=w329:errorcluster)  [unwired: 15 in, 1 out]
      }
      frame "Auto Align" {
        n141 = Unbundle By Name(w338) -> ("SA VISA"=w336:refnum<visa-resource-name>)
        n142 = case shown="True" "Auto Align Enable" {
          tunnel: w337 -> [w339 w344]
          tunnel: w336 -> [_ w345]
          tunnel: [w339 w341] -> w334
          frame False {
          }
          frame True {
            n143 = call <vilib>:"Set Busy.vi"("error in (no error)"=w344) -> ("error out"=w343:errorcluster)  [unwired: 9 in, 1 out]
            n144 = call "SpecAn Calibrate Set.vi"("error in (no error)"=w343, "VISA resource name"=w345) -> ("error out"=w342:errorcluster)  [unwired: 6 in, 3 out]
            n145 = local write "State"("Alignment In Progress" ("State")) -> ()
            n146 = call <vilib>:"Unset Busy.vi"("error in (no error)"=w342) -> ("error out"=w341:errorcluster)  [unwired: 10 in]
          }
        }
      }
      frame "TimeOut", Default {
        n147 = case shown="True" "Cont Update" {
          tunnel: w349 -> [w352 w355]
          tunnel: [w352 w354] -> w348
          tunnel: w347 -> [_ w353]
          frame False {
          }
          frame True {
            n148 = call "Queue Add Events to Back.vi"("Queue In"=w353, "State Array"=cluster{"State":string}[] [{"State"="Capture"}], "Error In"=w355) -> ("Error Out"=w354:errorcluster)  [unwired: 11 in, 1 out]
          }
        }
      }
      frame "Close Sessions" {
        n149 = Unbundle By Name(w361) -> ("SA VISA"=w357:refnum<visa-resource-name>)
        n150 = VISA Close(VISA resource name=w357, error in (no error)=w360) -> (error out=w358:errorcluster)
      }
      frame "Close GUI" {
      }
    }
    n151 = call "Error Manager.vi"("Error In"=w82) -> ("Error Out"=w83:errorcluster)  [unwired: 18 in]
  }
  "Error Out" <- w8
  n152 = flat-sequence {
    tunnel: w9 -> [_]
    tunnel: w8 -> [_]
    tunnel: w6 -> [w367]
    frame #0 {
      n153 = property class="App"() -> ("App.Kind"=w365:T7)  [unwired: 2 in, 2 out]
      n154 = Release Queue(queue=w367, force destroy? (F)=TRUE) -> (error out=w366:errorcluster)  [unwired: 1 in, 2 out]
      n155 = case shown="\"Run Time System\"" w365 {
        tunnel: w366 -> [w369 _]
        frame "Run Time System" {
          n156 = property class="VI"(error in=w369, "FP.State"=T6."Closed" ("Front Panel Window:State")) -> ()  [unwired: 1 in, 2 out]
        }
        frame "Development System", Default {
        }
      }
    }
  }
